vi "Module Configuration.vi"(8 "error in (no error)":errorcluster, 10 "Configuration":T1, 11 "Module ID":i32=-1) -> (0 "error out":errorcluster)   [LabVIEW 2014, in "Configurable.lvlib"]
doc: "_____\nCreated using Delacor QMH Event Scripter 4.0.0.68."
uses:
  Configurable.lvlib
  ModuleConfiguration--Cluster.ctl
  Module Configuration Argument--cluster.ctl
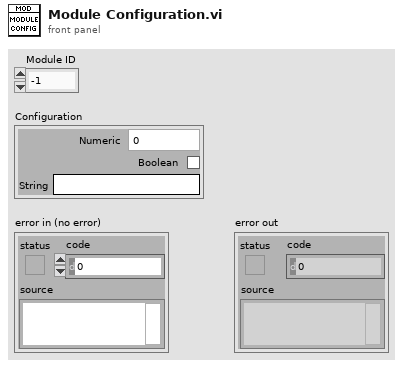
[diagram p1: front panel]
types:
  T1 = typedef "Configurable.lvlib/ModuleConfiguration--Cluster.ctl" = cluster{"Numeric":dbl, "Boolean":bool, "String":string}
  T2 = typedef "Configurable.lvlib/Module Configuration Argument--cluster.ctl" = cluster{"Module ID":i32, "Configuration":T1}
  T3 = typedef "Configurable.lvlib/Broadcast Events--cluster.ctl" = cluster{"Module Did Init":refnum<user-event>, "Status Updated":refnum<user-event>, "Error Reported":refnum<user-event>, "Module Did Stop":refnum<user-event>, "Update Module Execution Status":refnum<user-event>, "Module Configuration":refnum<user-event>}
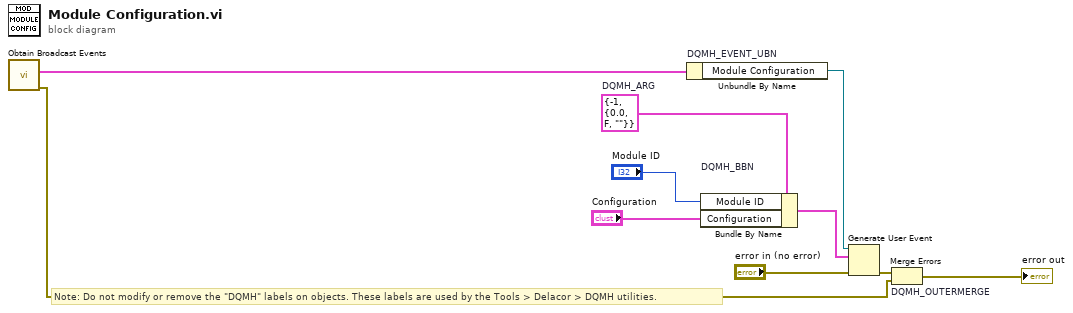
[diagram p0: block diagram]
diagram:
  w5 = T2 {"Module ID"=-1, "Configuration"={"Numeric"=0.0, "Boolean"=FALSE, "String"=""}}  # DQMH_ARG
  # "Note: Do not modify or remove the \"DQMH\" labels on objects. These labels are used by the Tools > Delacor > DQMH utilities."
  n1 = call "Obtain Broadcast Events.vi"() -> ("error out"=w2:errorcluster, "Configurable Broadcast Events"=w1:T3)  [unwired: 10 in]
  n2 = Unbundle By Name "DQMH_EVENT_UBN"(w1) -> ("Module Configuration"=w7:refnum<user-event>)
  n3 = Bundle By Name "DQMH_BBN"(cluster=w5, "Module ID"="Module ID", "Configuration"="Configuration") -> (w8:T2)
  n4 = Generate User Event(user event=w7, event data cluster=w8, error in="error in (no error)") -> (error out=w6:errorcluster)  [unwired: 1 in, 1 out]
  n5 = Merge Errors "DQMH_OUTERMERGE"(w6, w2) -> (→"error out":errorcluster)
